vi "5SecondTiming_BlinkingLEDand_TemperatureRise.vi"() -> ()   [LabVIEW 2019]
panel:
  out "Thermometer":i32(slide) scale=0.0..110.0
  out "Boolean":bool
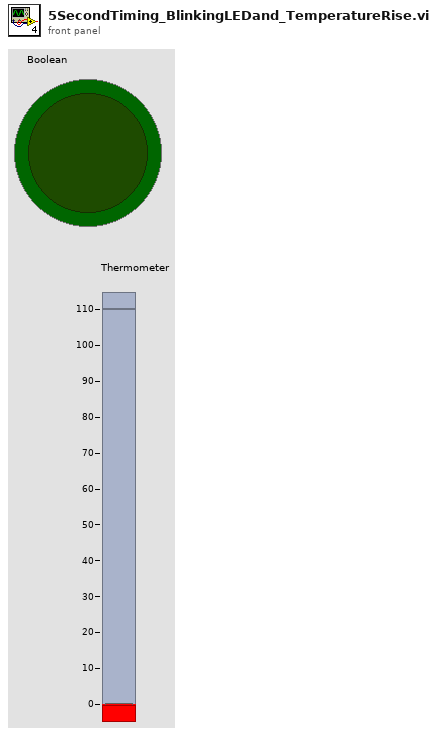
[diagram p1: front panel]
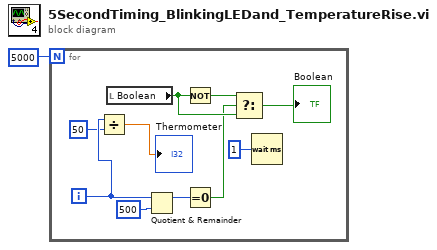
[diagram p0: block diagram]
diagram:
  n1 = for {
    N: 5000 -> [_]
    i -> [w4]
    n2 = Divide(x=w4, y=50) -> (x/y=→"Thermometer":dbl)
    n3 = local read "Boolean"() -> (w9:bool)
    n4 = Quotient & Remainder(x=w4, y=500) -> (x-y*floor(x/y)=w6:i32)  [unwired: 1 out]
    n5 = Not(x=w9) -> (.not. x?=w10:bool)
    n6 = Equal To 0?(x=w6) -> (x = 0?=w5:bool)
    n7 = Select(t=w10, s=w5, f=w9) -> (s? t:f=→"Boolean":bool)
    n8 = Wait (ms)(milliseconds to wait=u32 1) -> ()  [unwired: 1 out]
  }
